vi "LOAD_SUBPANEL.vi"(0 "SubPanel in":refnum<vi>, 3 "error in (no error)":errorcluster, 4 "VI Ref":refnum<vi>) -> (10 "error out":errorcluster)   [LabVIEW 2022 SP3]
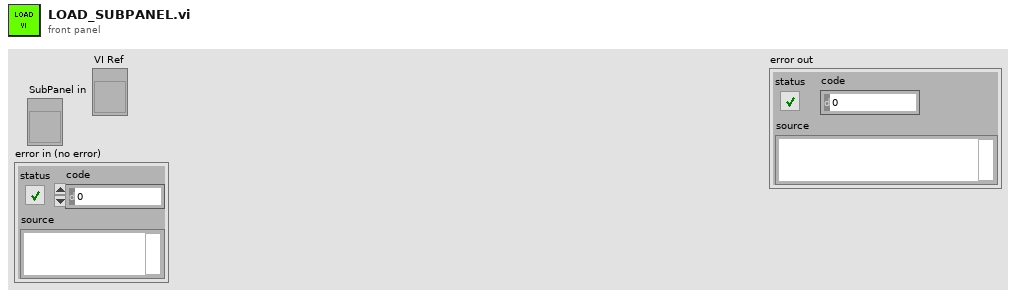
[diagram p1: front panel]
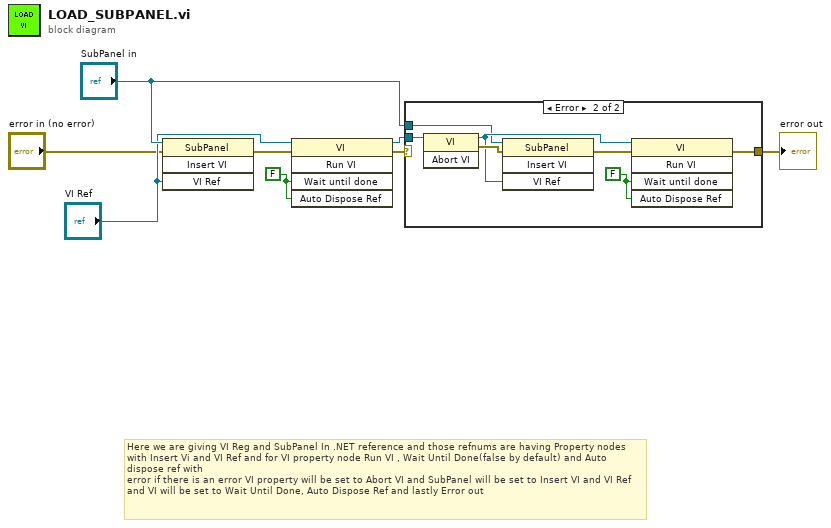
[diagram p0: block diagram]
diagram:
  w3 = FALSE ("Wait Until Done")
  # "Here we are giving VI Reg and SubPanel In .NET reference and those refnums are having Property nodes with Insert Vi and VI Ref and for VI property node Run VI , Wait Until Done(false by default) and Auto dispose ref with \nerror if there is an error VI property will be set to Abort VI and SubPanel will be set to Insert VI and VI Ref and VI will be set to Wait Until Done, Auto Dispose Ref and lastly Error out"
  n1 = invoke on="Invoke Node" class="SubPanel" method="Insert VI"(reference="SubPanel in", error in="error in (no error)", "VI Ref"="VI Ref") -> (error out=w6:errorcluster)  [unwired: 1 in, 3 out]
  n2 = invoke class="VI" method="Run VI"(reference="VI Ref", error in=w6, "Wait until done"=w3, "Auto Dispose Ref"=w3) -> (reference out=w8:refnum<vi>, error out=w7:errorcluster)  [unwired: 1 in, 3 out]
  n3 = case shown="Error" w7 {
    selector: w7 -> [w9 _]
    tunnel: w8 -> [_ w16]
    tunnel: "SubPanel in" -> [_ w11]
    tunnel: [w9 w10] -> w4
    frame No Error {
    }
    frame Error {
      w15 = FALSE ("Wait Until Done")
      n4 = invoke class="VI" method="Abort VI"(reference=w16) -> (reference out=w12:refnum<vi>, error out=w14:errorcluster)  [unwired: 2 in, 1 out]
      n5 = invoke on="Invoke Node" class="SubPanel" method="Insert VI"(reference=w11, error in=w14, "VI Ref"=w12) -> (error out=w13:errorcluster)  [unwired: 1 in, 3 out]
      n6 = invoke class="VI" method="Run VI"(reference=w12, error in=w13, "Wait until done"=w15, "Auto Dispose Ref"=w15) -> (error out=w10:errorcluster)  [unwired: 1 in, 4 out]
    }
  }
  "error out" <- w4
